vi "SCMain.vi"(0 "once?":bool, 1 "continousSequencer?":bool) -> ()   [LabVIEW 2014]
uses:
  <vilib>/Platform/TimedLoop/XDataNode/timing_clust.ctl
  <vilib>/Platform/TimedLoop/XDataNode/nitl_modes.ctl
  <vilib>/Platform/TimedLoop/XDataNode/wakeup.ctl
  SCGlobVars.vi
  <vilib>/rvi/Emulation/niFpgaSctlEmulationGetInTimedLoop.vi
  <vilib>/rvi/Emulation/niFpgaEmulationReportErrorSimple.vi
  <vilib>/rvi/Emulation/niFpgaGetClockAttributes.vi
  <vilib>/rvi/Emulation/niFpgaCriticalErrorInLSC.vi
  <vilib>/rvi/eio/common/nirviEmuTemplateMethod_errors.vi
  <vilib>/Platform/TimedLoop/XDataNode/XDataNode.xnode
  <vilib>/eio/EIONode/EIONode.xnode
  <vilib>/Platform/TimedLoop/XDataNode/XDNodeRunTimeDep.lvlib
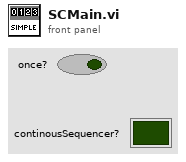
[diagram p1: front panel]
types:
  T1 = typedef "XDNodeRunTimeDep.lvlib/timing_clust.ctl" = cluster{"Expected End [f-1]":u64, "Actual End [f-1]":u64, "Finished Late? [f-1]":bool, "Expected End [i-1]":u64, "Actual End [i-1]":u64, "Finished Late? [i-1]":bool, "Expected Start [i]":u64, "Actual Start [i]":u64, "Expected Start [f]":u64, "Actual Start [f]":u64, "Source Name":string, "Structure Name":string, "Period":i64, "Deadline":i64, "Offset":i64, "Start":i64, "Priority":i32, "Timeout":i32, "Mode":T2, "Wakeup Reason":T3, "Error":errorcluster, "Source Type":string, "Secondary Source Type":string, "Global End Time":u64, "Global Start Time":u64, "Frame Duration":u64, "Iteration Duration":u64, "Assigned CPU":i32, "I/O Scan Engine Mode":u32}
  T2 = typedef "XDNodeRunTimeDep.lvlib/nitl_modes.ctl" = enum32{"No Change", "Process missed periods, maintain original phase", "Discard missed periods, maintain original phase", "Process missed periods, ignore original phase", "Discard missed periods, ignore original phase"}
  T3 = typedef "XDNodeRunTimeDep.lvlib/wakeup.ctl" = enum32{"Normal", "Aborted", "Asynchronous wakeup", "Timing source error", "Timed loop error", "Timeout"}
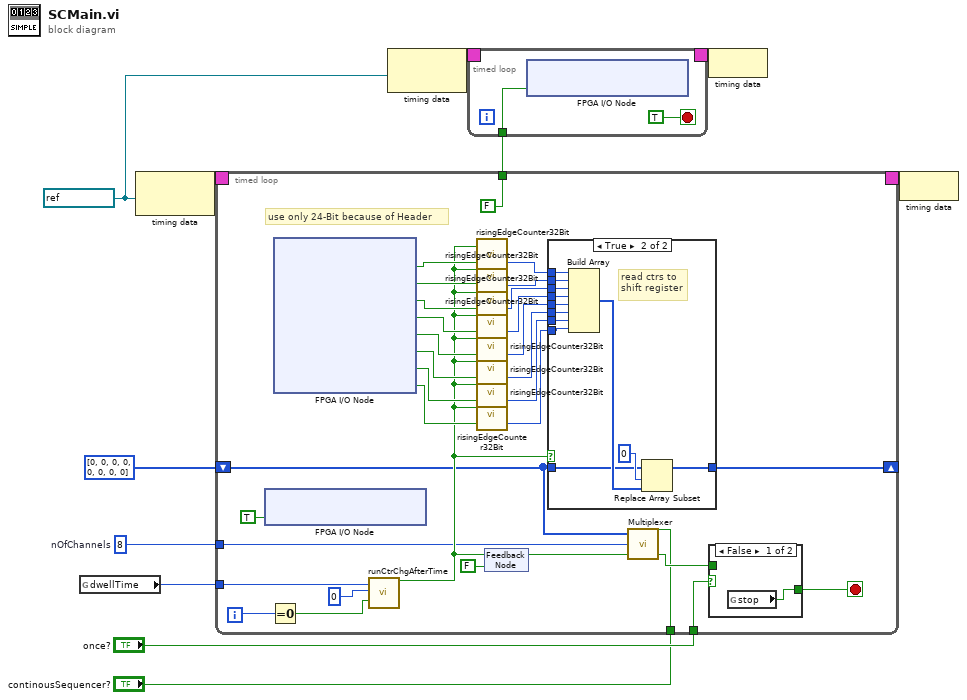
[diagram p0: block diagram]
diagram:
  w8 = u8 8  # nOfChannels
  w5 = refnum<k21> "100MHz" ("Source Name")
  n1 = global read "SCGlobVars.vi" "dwellTime"() -> (w2:u32)
  n2 = node-c288(w5) -> (w11:T1)
  n3 = timed-loop {
    timing: w11 -> [_]
    timing-out: [_] -> w10
    shift-right: [w27] -> _
    shift-left: u32[] [0, 0, 0, 0, 0, 0, 0, 0] -> [w23]
    tunnel: w8 -> [w21]
    tunnel: w2 -> [w26]
    tunnel: [FALSE ("SPScanFlagDio11Con1")] -> w4
    tunnel: "once?" -> [w16]
    tunnel: "continousSequencer?" -> [w15]
    i -> [w14]
    stop <- w17 stop-if-true
    # "use only 24-Bit because of Header"
    n4 = xnode "FPGA I/O Node"("SPScanFlagDio11Con1"=TRUE) -> ()  [unwired: 1 in, 1 out]
    n5 = Equal To 0?(x=w14) -> (x = 0?=w13:bool)
    n6 = xnode "FPGA I/O Node"() -> ("Connector1/DIO32"=w43:bool, "Connector1/DIO33"=w42:bool, "Connector1/DIO34"=w41:bool, "Connector1/DIO35"=w40:bool, "Connector1/DIO36"=w39:bool, "Connector1/DIO37"=w38:bool, "Connector1/DIO38"=w37:bool, "Connector1/DIO39"=w36:bool)  [unwired: 8 in, 8 out]
    n7 = call "runCtrChgAfterTime.vi"("timeDif(ticks)"=w26, "init(ticks)"=u32 0, "forceReset"=w13) -> ("change"=w25:bool)  [unwired: 16 in]
    n8 = call "risingEdgeCounter32Bit.vi"("In"=w43, "Reset"=w25) -> ("32BitCounter"=w35:u32)  [unwired: 1 in]
    n9 = call "risingEdgeCounter32Bit.vi"("In"=w42, "Reset"=w25) -> ("32BitCounter"=w34:u32)  [unwired: 1 in]
    n10 = call "risingEdgeCounter32Bit.vi"("In"=w41, "Reset"=w25) -> ("32BitCounter"=w33:u32)  [unwired: 1 in]
    n11 = call "risingEdgeCounter32Bit.vi"("In"=w40, "Reset"=w25) -> ("32BitCounter"=w32:u32)  [unwired: 1 in]
    n12 = call "risingEdgeCounter32Bit.vi"("In"=w39, "Reset"=w25) -> ("32BitCounter"=w31:u32)  [unwired: 1 in]
    n13 = call "risingEdgeCounter32Bit.vi"("In"=w38, "Reset"=w25) -> ("32BitCounter"=w30:u32)  [unwired: 1 in]
    n14 = call "risingEdgeCounter32Bit.vi"("In"=w37, "Reset"=w25) -> ("32BitCounter"=w29:u32)  [unwired: 1 in]
    n15 = call "risingEdgeCounter32Bit.vi"("In"=w36, "Reset"=w25) -> ("32BitCounter"=w28:u32)  [unwired: 1 in]
    n16 = feedback-in #1(w25) -> ()
    n17 = feedback #1(FALSE ("change")) -> (w22:bool)
    n18 = case shown="True" w25 {
      tunnel: w35 -> [_ w58]
      tunnel: w34 -> [_ w57]
      tunnel: w33 -> [_ w56]
      tunnel: w32 -> [_ w55]
      tunnel: w31 -> [_ w54]
      tunnel: w30 -> [_ w53]
      tunnel: w29 -> [_ w52]
      tunnel: w28 -> [_ w51]
      tunnel: [w46 w48] -> w27
      tunnel: w23 -> [w46 w47]
      frame False {
      }
      frame True {
        # "read ctrs to\nshift register"
        n19 = Build Array(w58, w57, w56, w55, w54, w53, w52, w51) -> (w50:u32[])
        n20 = Replace Array Subset(array=w47, new element=w50, index=0) -> (w48:u32[])
      }
    }
    n21 = call "Multiplexer.vi"("continousSequencer?"=w15, "write"=w22, "nOfChannels"=w21, "Data"=w23) -> ("done"=w18:bool)  [unwired: 1 in]
    n22 = case shown="False" w16 {
      tunnel: w18 -> [_ w45]
      tunnel: [w44 w45] -> w17
      frame False {
        n23 = global read "SCGlobVars.vi" "stop"() -> (w44:bool)
      }
      frame True {
      }
    }
  }
  n24 = node-c288(w5) -> (w7:T1)
  n25 = timed-loop {
    timing: w7 -> [_]
    timing-out: [_] -> w6
    tunnel: w4 -> [w61]
    stop <- TRUE stop-if-true
    n26 = xnode "FPGA I/O Node"("SPScanFlagDio11Con1"=w61) -> ()  [unwired: 1 in, 1 out]
  }
  n27 = node-c288(w6) -> ()
  n28 = node-c288(w10) -> ()
